vi "Main.vi"() -> ()   [LabVIEW 2011]
uses:
  <vilib>/gmath/NI_Gmath.lvlib
panel:
  out "Pres Linear Squared":cluster{"Y":dbl[], "Y":dbl[]}[](graph)
  out "Pres Transform":cluster{"Y":dbl[], "Y":dbl[]}[](graph)
  out "Pres Linearized":cluster{"Y":dbl[], "Y":dbl[]}[](graph)
  out "Bell Linearized":cluster{"Y":dbl[], "Y":dbl[]}[](graph)
  out "Y subarray":dbl[](array[numeric])
  out "X subarray":dbl[](array[numeric])
  out "Victor Empirical Data":cluster{"Y":dbl[], "Y":dbl[]}[](graph)
  out "Victor Empirical Data":dbl[][](array[numeric])
  out "Bell Transform":cluster{"Y":dbl[], "Y":dbl[]}[](graph)
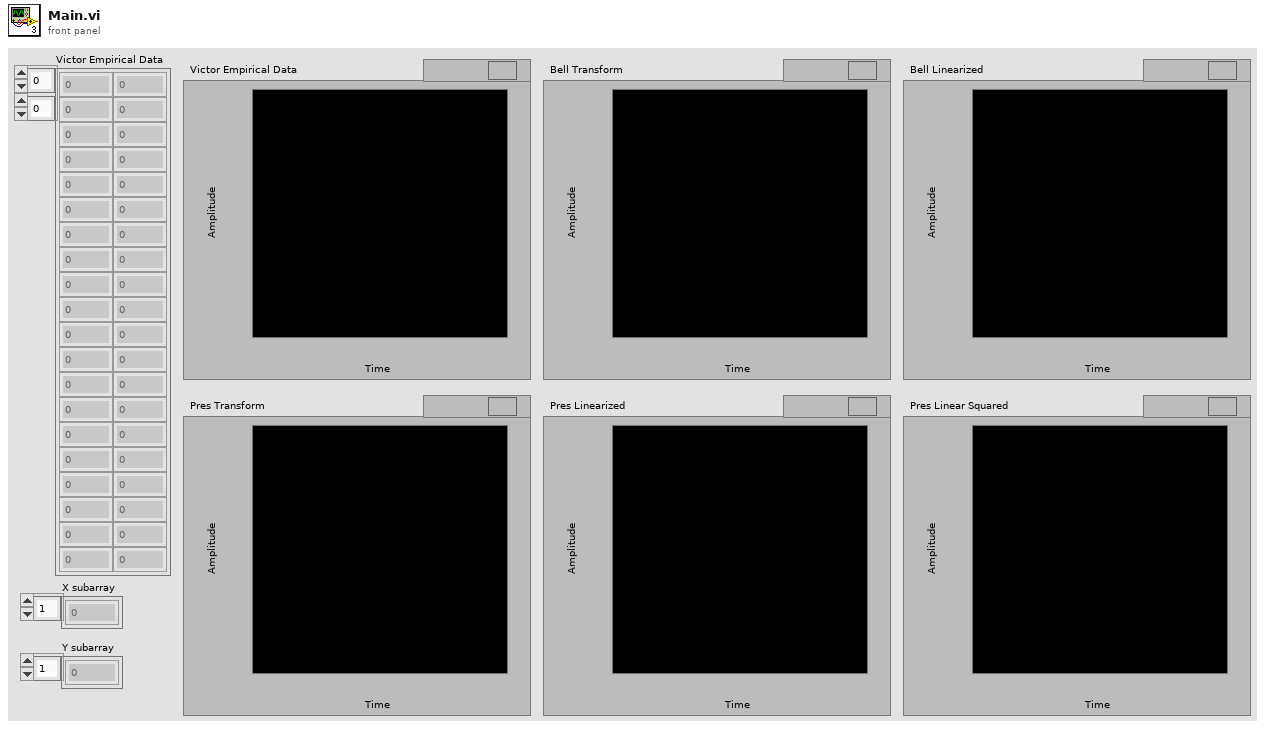
[diagram p1: front panel]
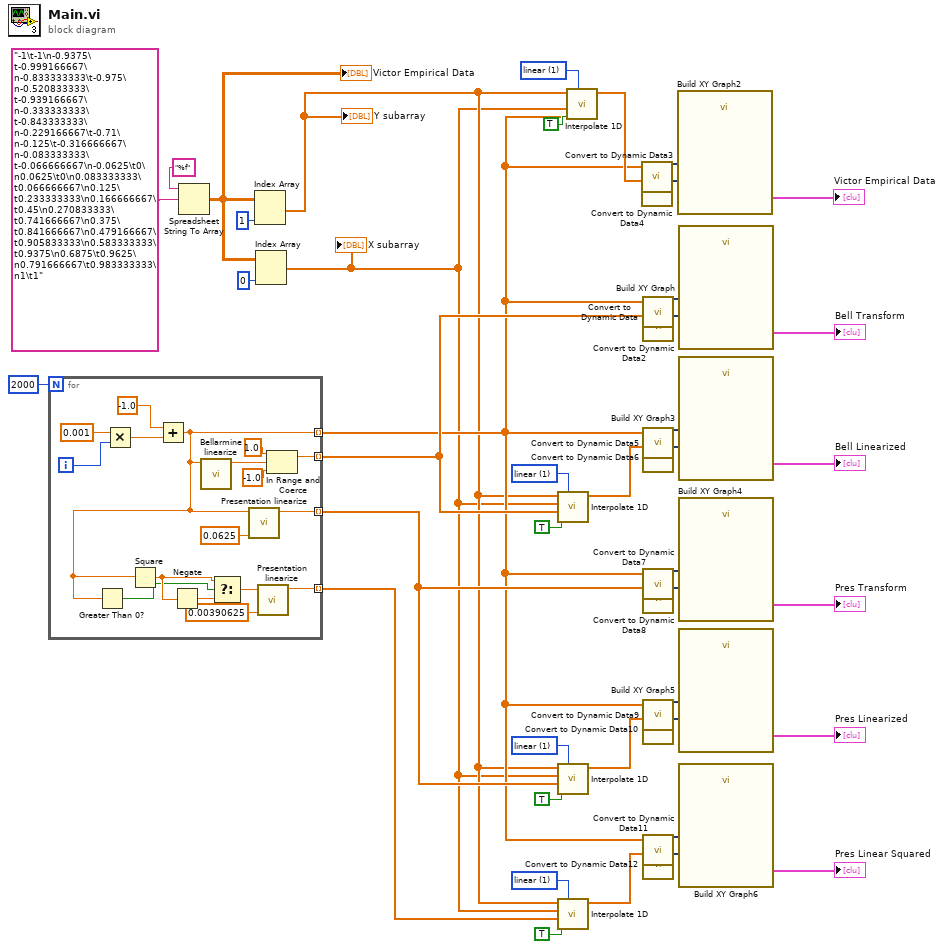
[diagram p0: block diagram]
diagram:
  w7 = 1 items=["nearest", "linear", "spline", "cubic Hermite", "Lagrange"] ("method")
  w18 = 1 items=["nearest", "linear", "spline", "cubic Hermite", "Lagrange"] ("method")
  w24 = 1 items=["nearest", "linear", "spline", "cubic Hermite", "Lagrange"] ("method")
  w33 = 1 items=["nearest", "linear", "spline", "cubic Hermite", "Lagrange"] ("method")
  n1 = for {
    N: 2000 -> [_]
    tunnel: [w51] -> w4 mode=indexing
    tunnel: [w45] -> w22 mode=indexing
    tunnel: [w55] -> w11 mode=indexing
    tunnel: [w48] -> w1 mode=indexing
    i -> [w56]
    n2 = Multiply(x=0.001, y=w56) -> (x*y=w57:dbl)
    n3 = Add(x=-1.0, y=w57) -> (x+y=w51:dbl)
    n4 = Greater Than 0?(x=w51) -> (x > 0?=w52:bool)
    n5 = Square(x=w51) -> (x^2=w53:dbl)
    n6 = Negate(x=w53) -> (-x=w54:dbl)
    n7 = call "Bellarmine linearize.vi"("Goal Speed"=w51) -> ("Output"=w46:dbl)  [unwired: 8 in]
    n8 = Select(t=w53, s=w52, f=w54) -> (s? t:f=w49:dbl)
    n9 = call "Presentation linearize.vi"("Deadband"=0.0625, "Input"=w51) -> ("Output"=w55:dbl)  [unwired: 9 in]
    n10 = call "Presentation linearize.vi"("Deadband"=0.00390625, "Input"=w49) -> ("Output"=w48:dbl)  [unwired: 9 in]
    n11 = In Range and Coerce(upper limit=1.0, x=w46, lower limit=-1.0) -> (coerced(x)=w45:dbl)  [unwired: 1 out]
  }
  n12 = Spreadsheet String To Array(format string="%f", spreadsheet string="-1\t-1\n-0.9375\t-0.999166667\n-0.833333333\t-0.975\n-0.520833333\t-0.939166667\n-0.333333333\t-0.843333333\n-0.229166667\t-0.71\n-0.125\t-0.316666667\n-0.083333333\t-0.066666667\n-0.0625\t0\n0.0625\t0\n0.083333333\t0.066666667\n0.125\t0.233333333\n0.166666667\t0.45\n0.270833333\t0.741666667\n0.375\t0.841666667\n0.479166667\t0.905833333\n0.583333333\t0.9375\n0.6875\t0.9625\n0.791666667\t0.983333333\n1\t1") -> (array=w35:dbl[][])  [unwired: 2 in]
  "Victor Empirical Data" <- w35
  n13 = Index Array(array=w35, index (col)=1 ("disabled index (col)")) -> (element=w3:dbl[])  [unwired: 1 in]
  "Y subarray" <- w3
  n14 = Index Array(array=w35, index (col)=0 ("disabled index (col)")) -> (element=w2:dbl[])  [unwired: 1 in]
  "X subarray" <- w2
  n15 = call <vilib>:"Interpolate 1D.vi"("method"=w24, "X is monotonic"=TRUE, "xi"=w22, "X"=w2, "Y"=w3) -> ("yi"=w21:dbl[])  [unwired: 4 in, 2 out]
  n16 = call <vilib>:"Interpolate 1D.vi"("method"=w18, "X is monotonic"=TRUE, "xi"=w11, "X"=w2, "Y"=w3) -> ("yi"=w20:dbl[])  [unwired: 4 in, 2 out]
  n17 = call <vilib>:"Interpolate 1D.vi"("method"=w7, "X is monotonic"=TRUE, "xi"=w1, "X"=w2, "Y"=w3) -> ("yi"=w5:dbl[])  [unwired: 4 in, 2 out]
  n18 = call <vilib>:"Interpolate 1D.vi"("method"=w33, "X is monotonic"=TRUE, "xi"=w4, "X"=w2, "Y"=w3) -> ("yi"=w28:dbl[])  [unwired: 4 in, 2 out]
  n19 = call "Convert to Dynamic Data3"("Array"=w4) -> ("Dynamic Data Type"=w30:dynamicdata)  [unwired: 3 in]
  n20 = call "Convert to Dynamic Data4"("Array"=w28) -> ("Dynamic Data Type"=w29:dynamicdata)  [unwired: 3 in]
  n21 = call "Convert to Dynamic Data"("Array"=w4) -> ("Dynamic Data Type"=w40:dynamicdata)  [unwired: 3 in]
  n22 = call "Convert to Dynamic Data2"("Array"=w22) -> ("Dynamic Data Type"=w39:dynamicdata)  [unwired: 3 in]
  n23 = call "Convert to Dynamic Data5"("Array"=w4) -> ("Dynamic Data Type"=w26:dynamicdata)  [unwired: 3 in]
  n24 = call "Convert to Dynamic Data6"("Array"=w21) -> ("Dynamic Data Type"=w27:dynamicdata)  [unwired: 3 in]
  n25 = call "Convert to Dynamic Data7"("Array"=w4) -> ("Dynamic Data Type"=w13:dynamicdata)  [unwired: 3 in]
  n26 = call "Convert to Dynamic Data8"("Array"=w11) -> ("Dynamic Data Type"=w14:dynamicdata)  [unwired: 3 in]
  n27 = call "Convert to Dynamic Data9"("Array"=w4) -> ("Dynamic Data Type"=w16:dynamicdata)  [unwired: 3 in]
  n28 = call "Convert to Dynamic Data10"("Array"=w20) -> ("Dynamic Data Type"=w15:dynamicdata)  [unwired: 3 in]
  n29 = call "Convert to Dynamic Data11"("Array"=w4) -> ("Dynamic Data Type"=w9:dynamicdata)  [unwired: 3 in]
  n30 = call "Convert to Dynamic Data12"("Array"=w5) -> ("Dynamic Data Type"=w10:dynamicdata)  [unwired: 3 in]
  n31 = call "Build XY Graph2"("Y Input"=w29, "X Input"=w30) -> ("XY Graph"=→"Victor Empirical Data":cluster{"Y":dbl[], "Y":dbl[]}[])  [unwired: 3 in, 6 out]
  n32 = call "Build XY Graph"("Y Input"=w39, "X Input"=w40) -> ("XY Graph"=→"Bell Transform":cluster{"Y":dbl[], "Y":dbl[]}[])  [unwired: 3 in, 6 out]
  n33 = call "Build XY Graph3"("Y Input"=w27, "X Input"=w26) -> ("XY Graph"=→"Bell Linearized":cluster{"Y":dbl[], "Y":dbl[]}[])  [unwired: 3 in, 6 out]
  n34 = call "Build XY Graph4"("Y Input"=w14, "X Input"=w13) -> ("XY Graph"=→"Pres Transform":cluster{"Y":dbl[], "Y":dbl[]}[])  [unwired: 3 in, 6 out]
  n35 = call "Build XY Graph5"("Y Input"=w15, "X Input"=w16) -> ("XY Graph"=→"Pres Linearized":cluster{"Y":dbl[], "Y":dbl[]}[])  [unwired: 3 in, 6 out]
  n36 = call "Build XY Graph6"("Y Input"=w10, "X Input"=w9) -> ("XY Graph"=→"Pres Linear Squared":cluster{"Y":dbl[], "Y":dbl[]}[])  [unwired: 3 in, 6 out]
